vi "DAQNavi Write (Analog Wfm 1Chan NSamp).vi"(8 "error in (no error)":errorcluster, 9 "timeout":dbl=10.0, 10 "data":waveform(dbl), 11 "task in":i32) -> (0 "error out":errorcluster, 2 "number of samples written per channel":u32, 3 "task out":i32)   [LabVIEW 2020]
uses:
  DAQNavi_LV.dll
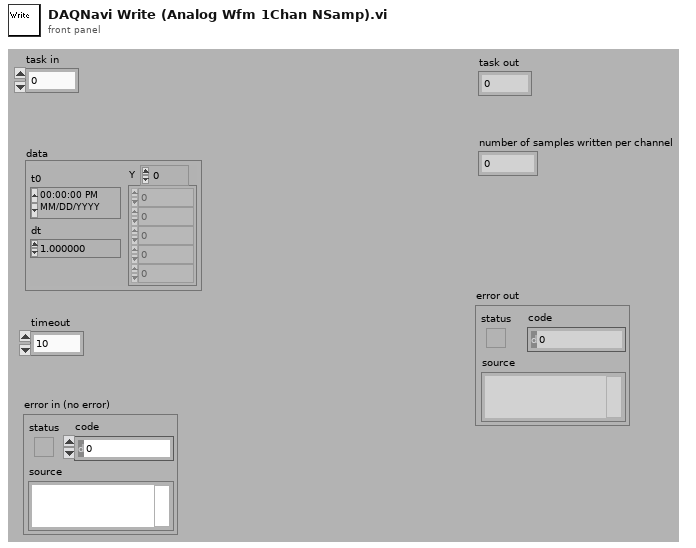
[diagram p1: front panel]
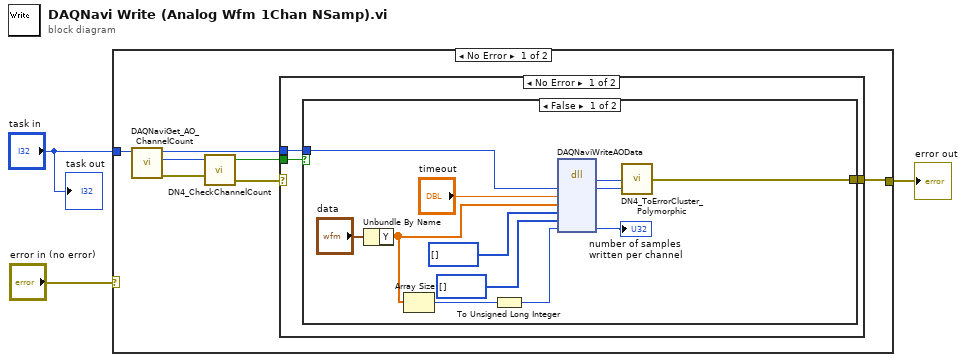
[diagram p0: block diagram]
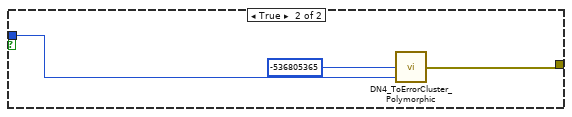
[diagram p2: hidden frame]
diagram:
  n1 = case shown="No Error" "error in (no error)" {
    selector: "error in (no error)" -> [_ w30]
    tunnel: [w9 w30] -> w2
    tunnel: "task in" -> [w10 _]
    frame No Error {
      n2 = call "DAQNaviGet_AO_ChannelCount.vi"("task in"=w10) -> ("error out"=w7:errorcluster, "channel count"=w8:i32, "task out"=w4:i32)  [unwired: 1 in, 7 out]
      n3 = call "DN4_CheckChannelCount.vi"("error out"=w7, "channel count"=w8) -> ("error IO"=w5:errorcluster, "greater than 1?"=w6:bool)  [unwired: 2 out]
      n4 = case shown="No Error" w5 {
        selector: w5 -> [_ w29]
        tunnel: w6 -> [w13 _]
        tunnel: w4 -> [w12 _]
        tunnel: [w11 w29] -> w9
        frame No Error {
          n5 = case shown="False" w13 {
            tunnel: [w19 w27] -> w11
            tunnel: w12 -> [w25 w26]
            frame False {
              n6 = Unbundle By Name("data") -> ("Y"=w17:dbl[])
              n7 = Array Size(array=w17) -> (size(s)=w16:i32)
              n8 = To Unsigned Long Integer(number=w16) -> (unsigned 32bit integer=w15:u32)
              n9 = dll-call lib="DAQNavi_LV.dll" fn="DAQNaviWriteAOData"("taskID"=w25, "timeout"="timeout", "scaledData"=w17, "rawData16"=u16[] [], "rawData32"=u32[] [], "samples"=w15) -> ("return type"=w20:i32, "taskID"=w14:i32, "samples"=→"number of samples written per channel":u32)  [unwired: 4 in, 5 out]
              n10 = call "DN4_ToErrorCluster_Polymorphic.vi"("task id"=w14, "error code"=w20) -> ("error out"=w19:errorcluster)  [unwired: 3 out]
            }
            frame True {
              n11 = call "DN4_ToErrorCluster_Polymorphic.vi"("task id"=w26, "error code"=-536805365 ("error code (0)")) -> ("error out"=w27:errorcluster)  [unwired: 3 out]
            }
          }
        }
        frame Error {
        }
      }
    }
    frame Error {
    }
  }
  "error out" <- w2
  "task out" <- "task in"
